vi "Check Message Path.vi"(8 "error in (no error)":errorcluster, 10 ".proto Path":path) -> (0 "error out":errorcluster, 2 "Starting Folder":path)   [LabVIEW 2020, in "LV-Protoc.lvlib" / "LV-Protoc.lvclass"]
uses:
  LV-Protoc.lvclass
  lv-cdm/CDM-Config/Config-JSON/Config-JSON.lvclass
  C:/dev/lv20CE/relink/lv-cdm/CDM-Config/Config Storage/Config Storage.lvclass
  LV-Protoc.lvclass/LV-Protoc.ctl
  lv-cdm/CDM-Config/Config Storage/Config Storage.lvclass
  lv-cdm/CDM-Config/Config Manager/Config Manager.lvclass
  lv-cdm/CDM-Config/Config Element/Config Element.lvclass
  lv-cdm/CDM-Config/CDM-Config.lvlib
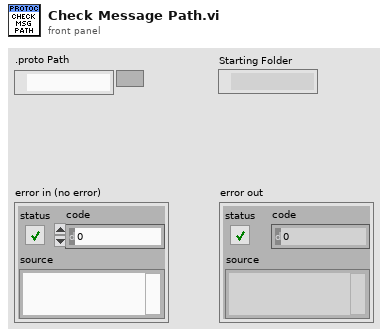
[diagram p1: front panel]
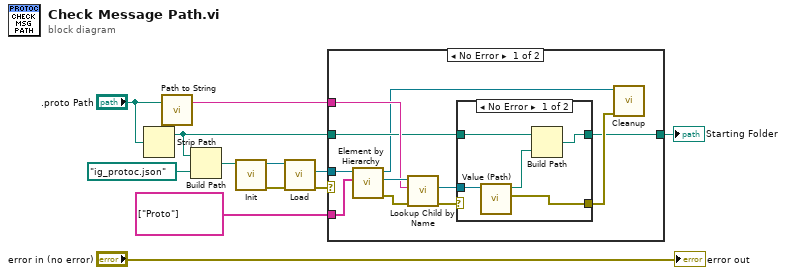
[diagram p0: block diagram]
diagram:
  n1 = Strip Path(path=".proto Path") -> (stripped path=w6:path)  [unwired: 1 out]
  n2 = call "Path to String.vi"("Path"=".proto Path") -> ("Path String"=w5:string)  [unwired: 2 in]
  n3 = Build Path(base path=w6, name or relative path=path "ig_protoc.json") -> (appended path=w11:path)
  n4 = call "Init.vi"("Path"=w11) -> ("error out"=w10:errorcluster, "Config-JSON out"=w9:refnum<class "Config-JSON.lvclass">)  [unwired: 9 in]
  n5 = call "Load.vi"("error in (no error)"=w10, "Config Storage in"=w9) -> ("error out"=w8:errorcluster, "Config"=w7:refnum<class "Config Manager.lvclass">)  [unwired: 7 in, 1 out]
  n6 = case shown="No Error" w8 {
    tunnel: w7 -> [w22 _]
    tunnel: w6 -> [w15 w31]
    tunnel: w5 -> [w18 _]
    tunnel: [w14 w31] -> w4
    tunnel: string[] ["Proto"] ("Hierarchy") -> [w21 _]
    frame No Error {
      n7 = call "Element by Hierarchy.vi"("Hierarchy"=w21, "Config Manager in"=w22) -> ("error out"=w19:errorcluster, "Config Element"=w20:refnum<class "Config Element.lvclass">, "Config Manager out"=w13:refnum<class "Config Manager.lvclass">)  [unwired: 7 in]
      n8 = call "Lookup Child by Name.vi"("error in (no error)"=w19, "Name"=w18, "Config Element in"=w20) -> ("error out"=w17:errorcluster, "Child"=w16:refnum<class "Config Element.lvclass">)  [unwired: 5 in, 2 out]
      n9 = case shown="No Error" w17 {
        selector: w17 -> [_ w29]
        tunnel: w16 -> [w28 _]
        tunnel: w15 -> [w27 w30]
        tunnel: [w25 w30] -> w14
        tunnel: [w24 w29] -> w23
        frame No Error {
          n10 = call "Value (Path).vi"("Config Element in"=w28) -> ("error out"=w24:errorcluster, "Path Value"=w26:path)  [unwired: 9 in]
          n11 = Build Path(base path=w27, name or relative path=w26) -> (appended path=w25:path)
        }
        frame Error {
          # "proto file entry does not exist yet"
        }
      }
      n12 = call "Cleanup.vi"("error in (no error)"=w23, "Config Manager in"=w13) -> ()  [unwired: 9 in, 1 out]
    }
    frame Error {
      # "Config for protoc does not exist in .proto folder yet."
    }
  }
  "Starting Folder" <- w4
  "error out" <- "error in (no error)"
